vi "SpectralCurrent.vi"() -> ()   [LabVIEW 2009]
uses:
  <vilib>/Utility/file.llb/Write To Spreadsheet File (DBL).vi
  <vilib>/DAQmx/configure/timing.llb/DAQmx Timing (Sample Clock).vi
  <vilib>/DAQmx/create/channels.llb/DAQmx Create Channel (AI-Voltage-Basic).vi
  <vilib>/Utility/file.llb/Read From Spreadsheet File (DBL).vi
  <vilib>/DAQmx/read.llb/DAQmx Read (Analog 1D DBL 1Chan NSamp).vi
  <vilib>/Analysis/NI_AALBase.lvlib
panel:
  in  "Open Power Normalization Values Path":path
  in  "Normalize with file?":bool
  in  "Power Values Path":path
  out "Normalized Current":cluster{dbl[], dbl[]}(graph)
  in  "Save Current Path":path
  in  "Save Current?":bool
  out "Spectral Current":cluster{dbl[], dbl[]}(graph)
  in  "End Scan":bool
  out "Measuring Current":bool
  in  "Current":tag
  in  "Current Scan":bool
  in  "Exit":bool
  out "Scanning":bool
  in  "Scan Save Path":path
  in  "Save Power Scan?":bool
  out "Power Scan":cluster{dbl[], dbl[]}(graph)
  in  "Abort\n Scan":bool
  in  "Wavelength\n   Step Size":dbl=1.0 min=0.1 max=100.0
  in  "Starting\nWavelength":dbl=400.0 min=400.0 max=2500.0
  in  "Ending\nWavelength":dbl=500.0 min=451.0 max=2501.0
  in  "Step Time (sec)":dbl=1.0 min=0.1 max=10.0 step=0.1
  in  "Measurement Save Path":path
  in  "Save Measurement?":bool
  out "Power Measurement":dbl[](graph)
  out "Readout value":dbl format="%^#_9e"
  out "Readout string":string
  in  "Timeout [ms]":i32=1000
  out "New":bool
  out "ZeroValue":dbl
  out "RANG_Val":dbl
  out "RANG_lbl":string
  out "Rng":string
  out "AUTO?":bool
  in  "AUTO":bool=TRUE
  in  "Range":i16=1 min=1 max=6 step=1
  out "PM Error log":string
  in  "Beam\nDiameter (mm)":dbl=4.0 min=1.0 max=9.0 step=0.5
  in  "BWIn":u16(ring) caption="Bandwidth" items=["HIGH", "LOW"]
  in  "Averaging Rate":i32=300 min=33 max=5000 step=1
  in  "Zero?":bool
  in  "Stop Measurement":bool
  out "IDN String":string
  out "Sensor SN":string
  out "Sensor Name":string
  out "Incrementing Down":bool
  out "Changing Wavelength":bool
  out "Incrementing Up":bool
  in  "Increment":dbl=10.0 min=0.1 max=50.0
  in  "Target\nWavelength":dbl=400.0 min=400.0 max=3000.0
  out "Wavelength (nm)":dbl
  out "Turning Turret":bool
  out "Current Blaze":string caption="Grating Blaze"
  out "Grating Density":dbl
  out "Grating Index":i32
  in  "Select Grating Blaze":string(combo)
  out "error out":errorcluster
  out "Status":string
  out "Emulating":bool
  out "Initialized":bool
  in  "Force\nInitialization":bool
  in  "Mono ID":string(combo)
  out "Current UniqueID":string
  in  "Measure Power":bool
  in  "Initialize":bool
  in  "Switch Turret":bool
  in  "Scan":bool
  in  "Increment Down":bool
  in  "Increment Up":bool
  in  "Change Wavelength":bool
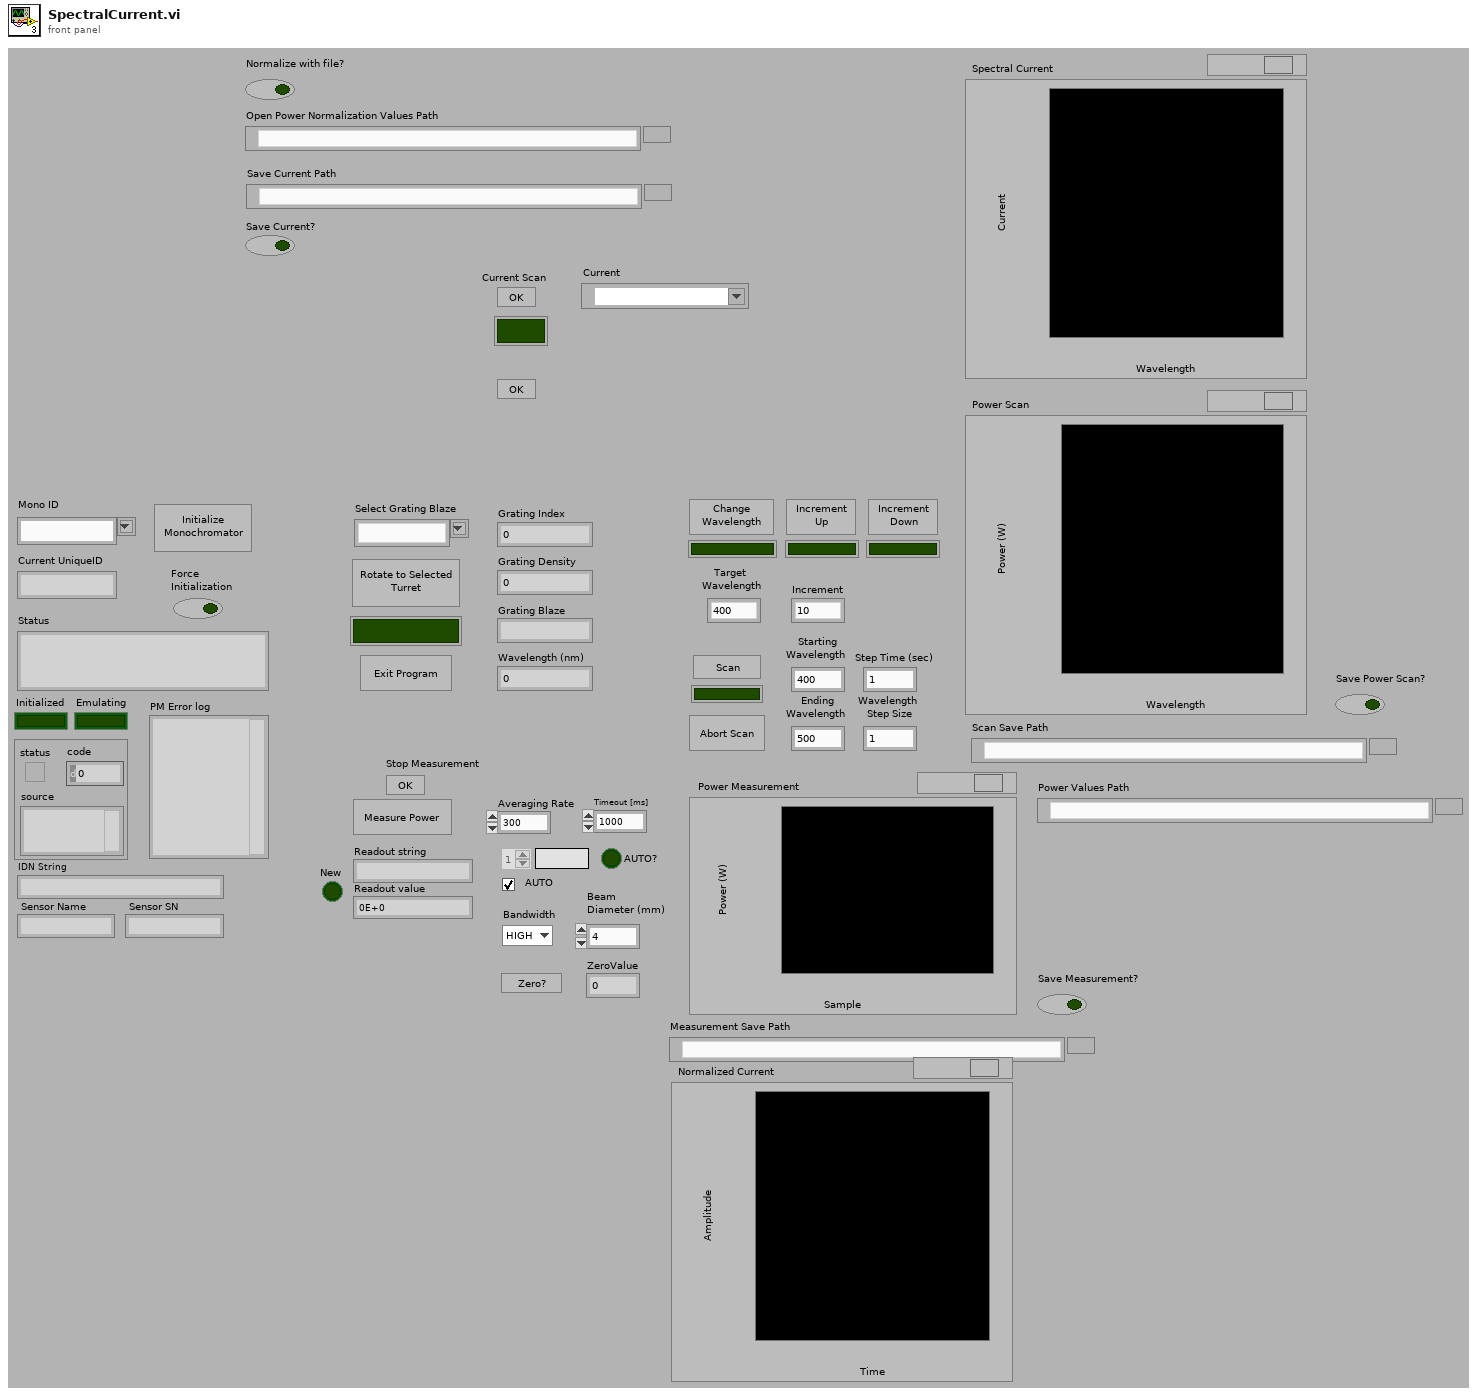
[diagram p1: front panel]
types:
  T1 = enum16{"0", "1", "2", "3", "4", "5", "6", "7", "8", "9"}
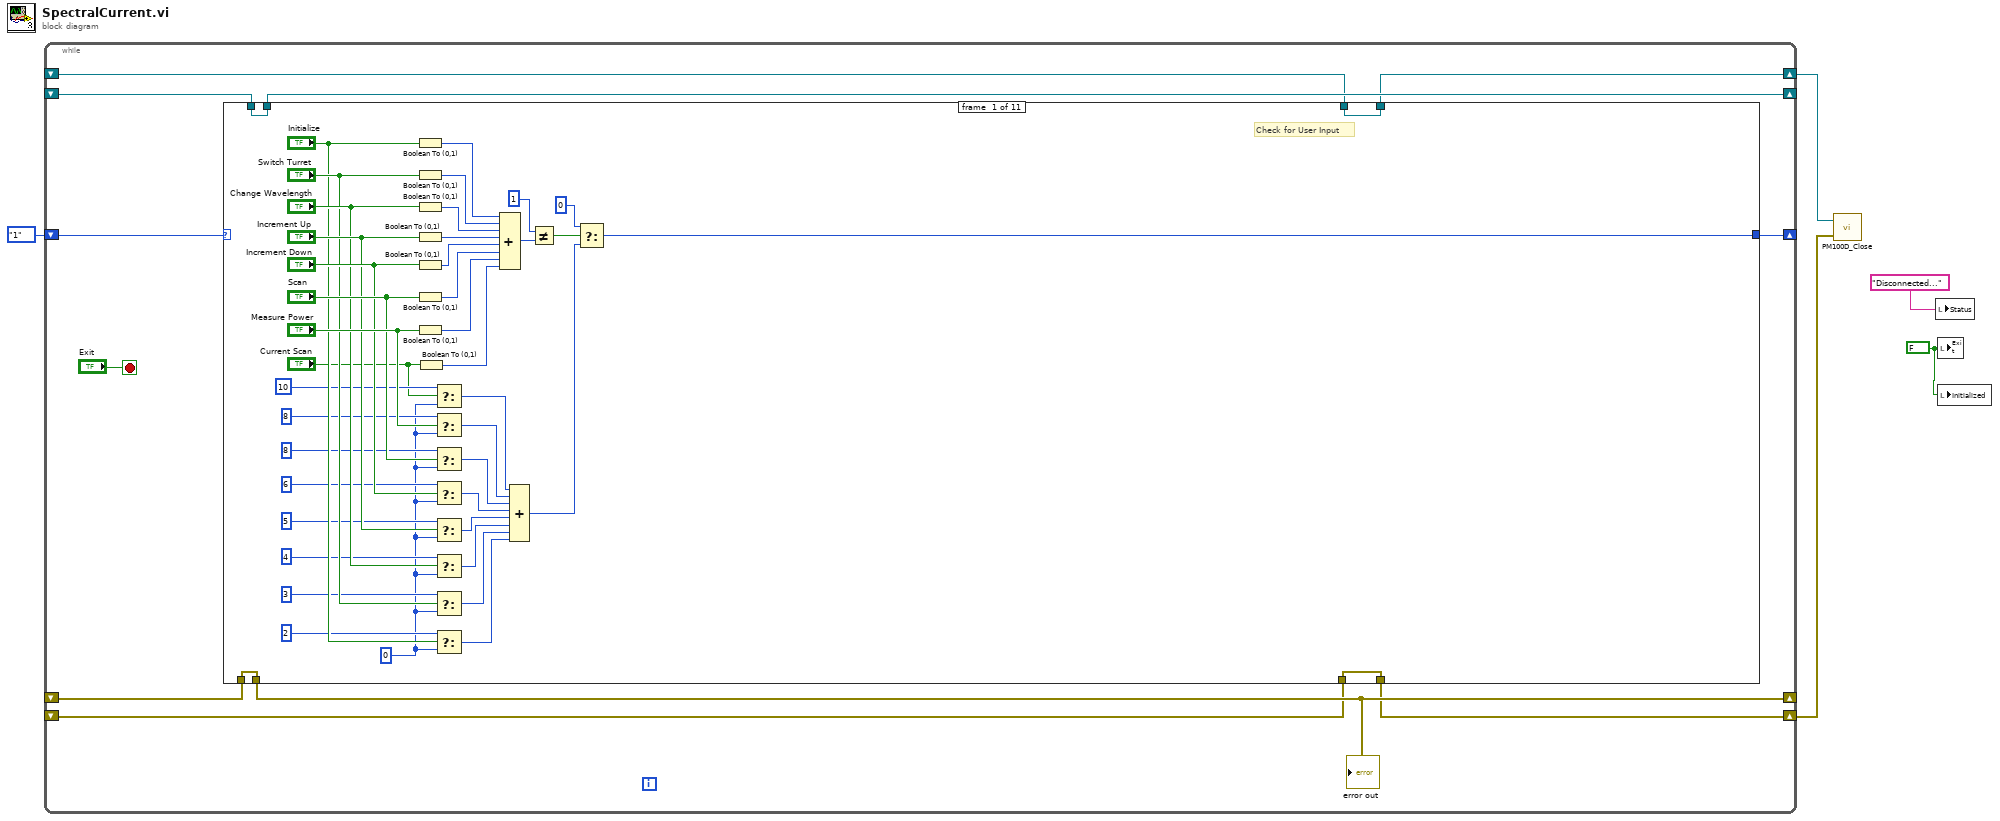
[diagram p0: block diagram]
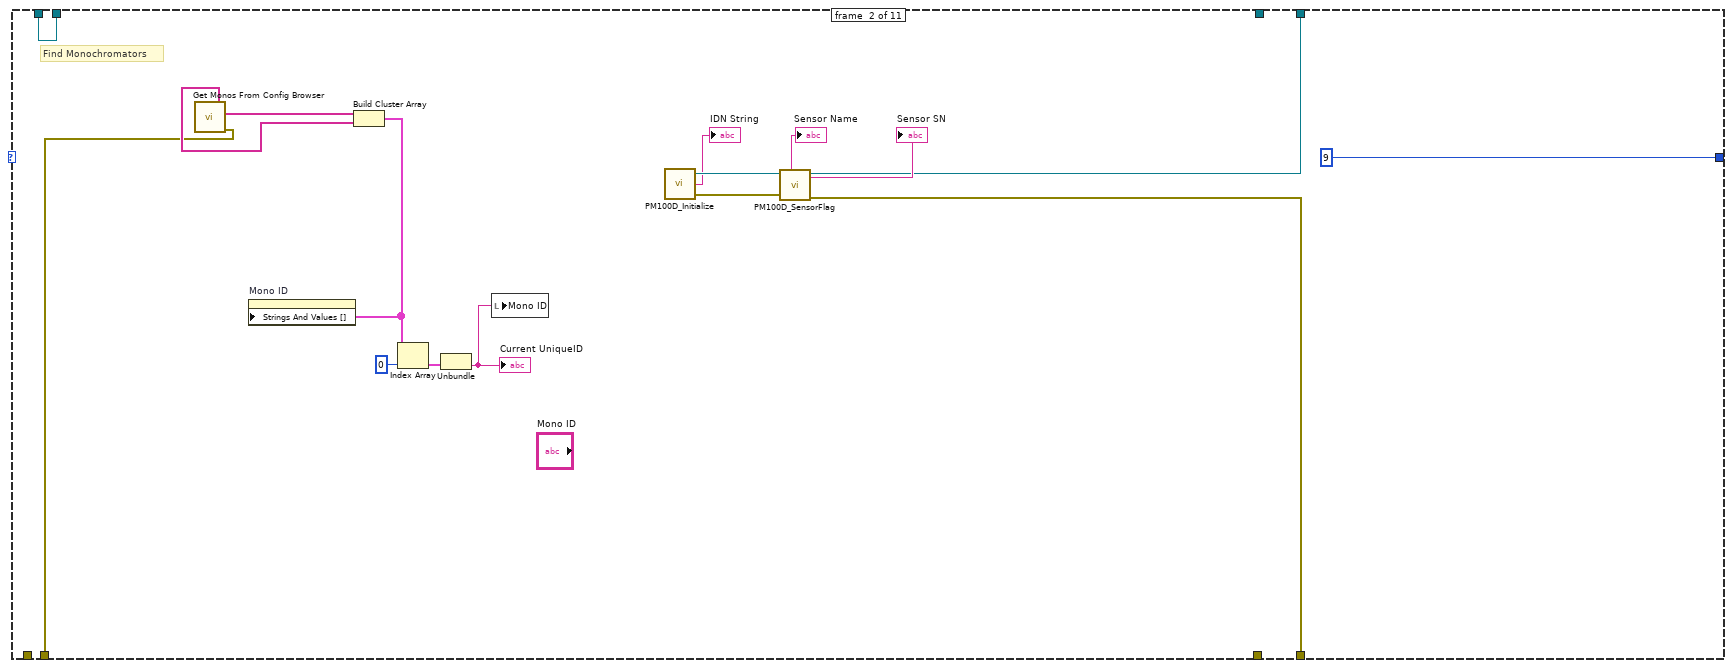
[diagram p2: hidden frame]
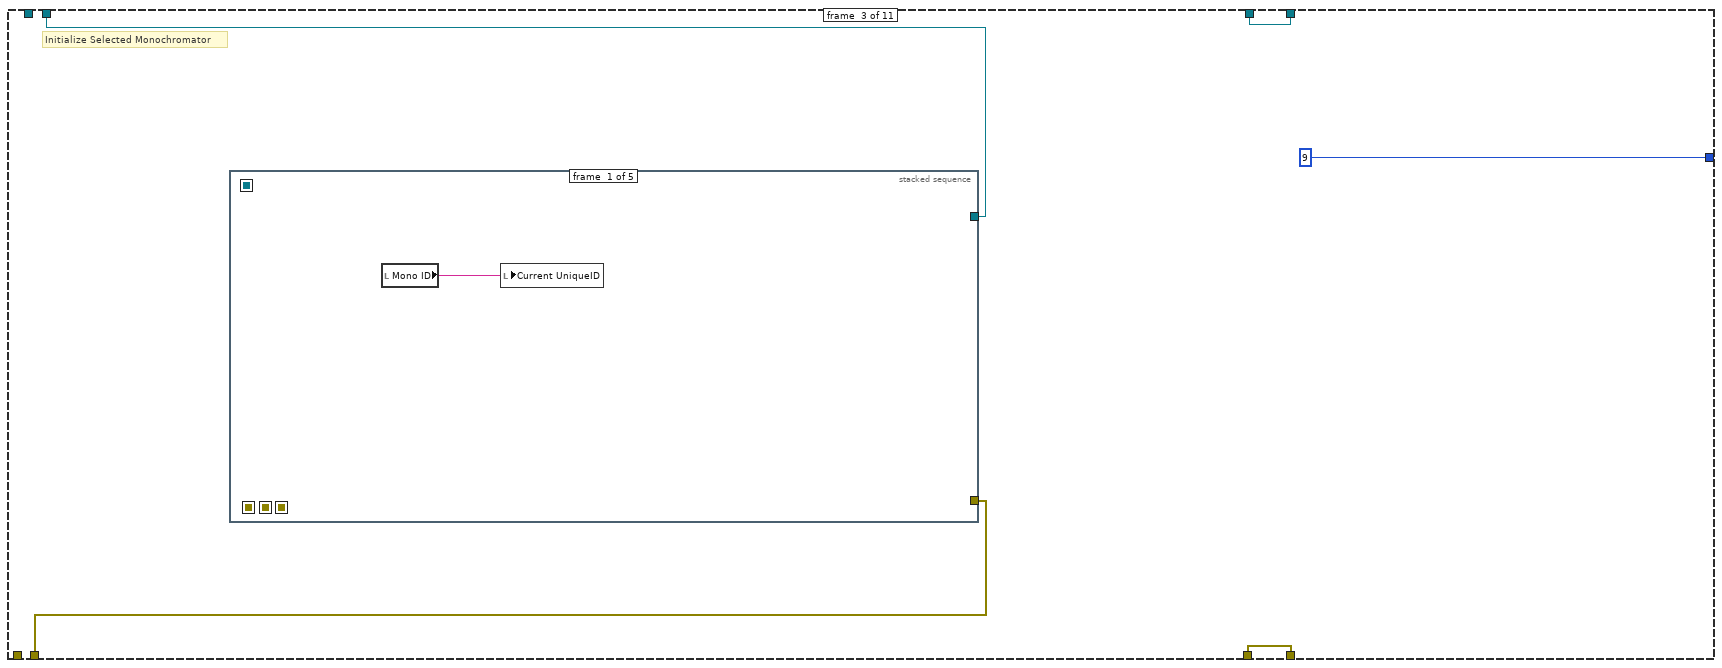
[diagram p3: hidden frame]
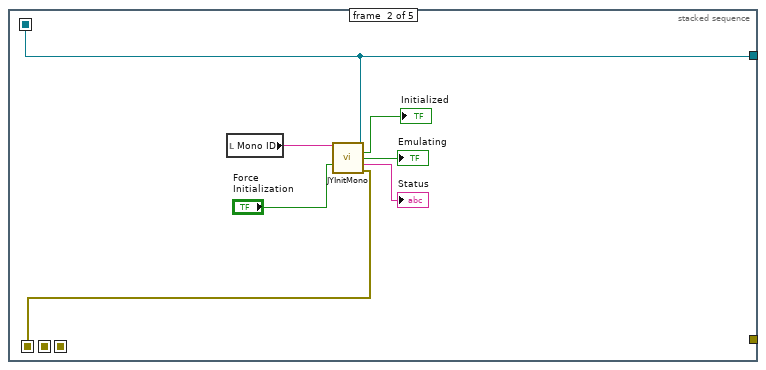
[diagram p4: hidden frame]
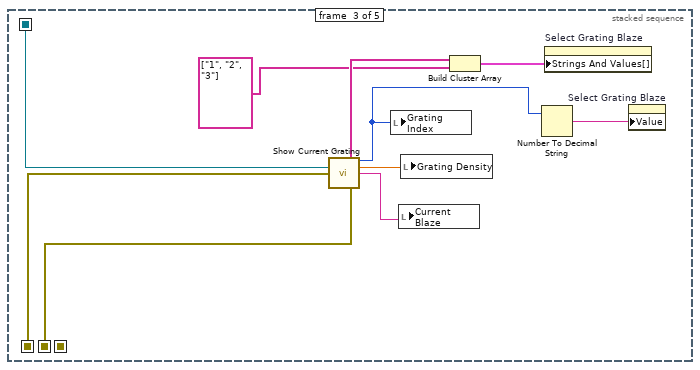
[diagram p5: hidden frame]
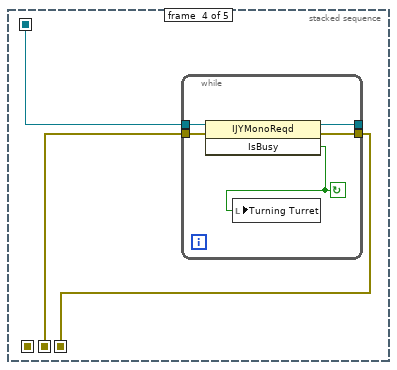
[diagram p6: hidden frame]
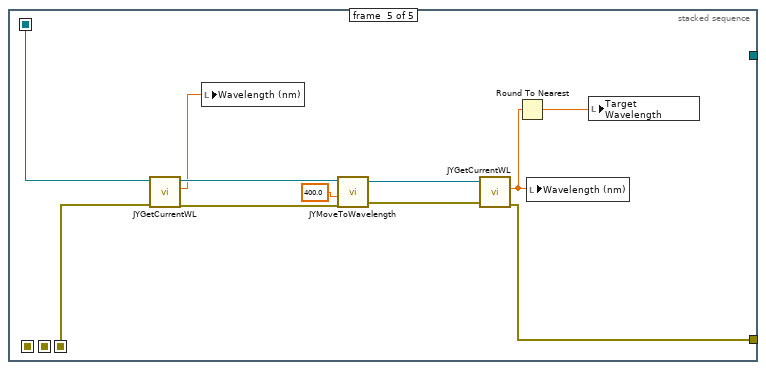
[diagram p7: hidden frame]
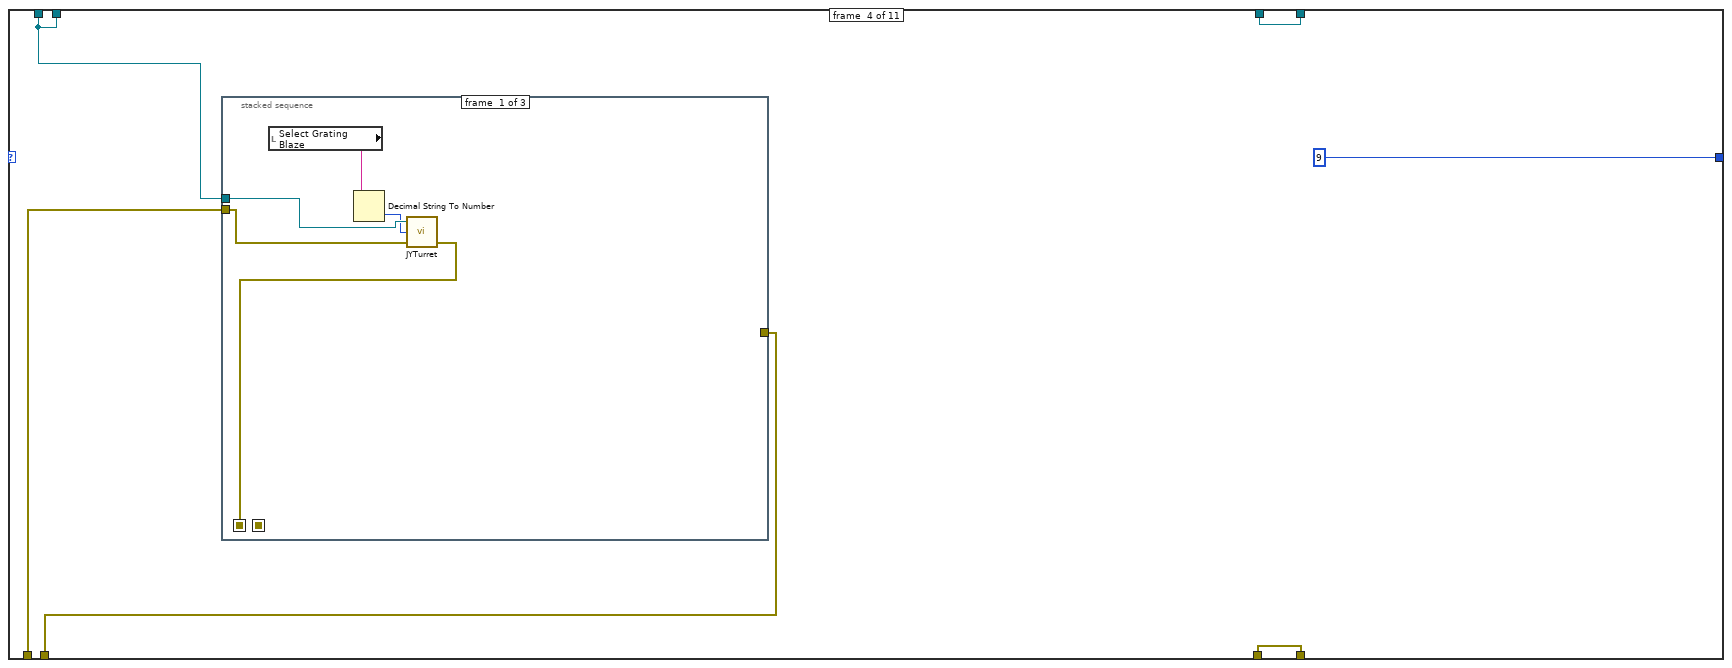
[diagram p8: hidden frame]
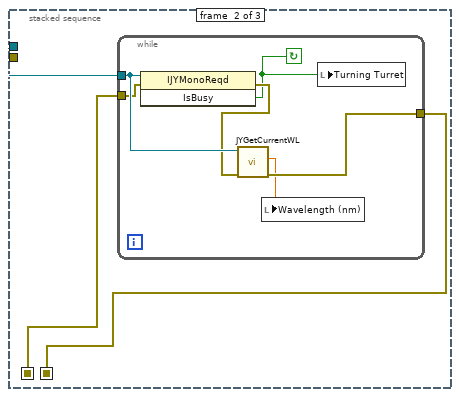
[diagram p9: hidden frame]
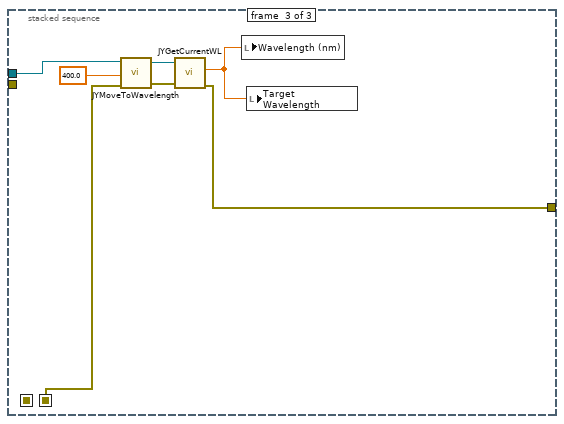
[diagram p10: hidden frame]
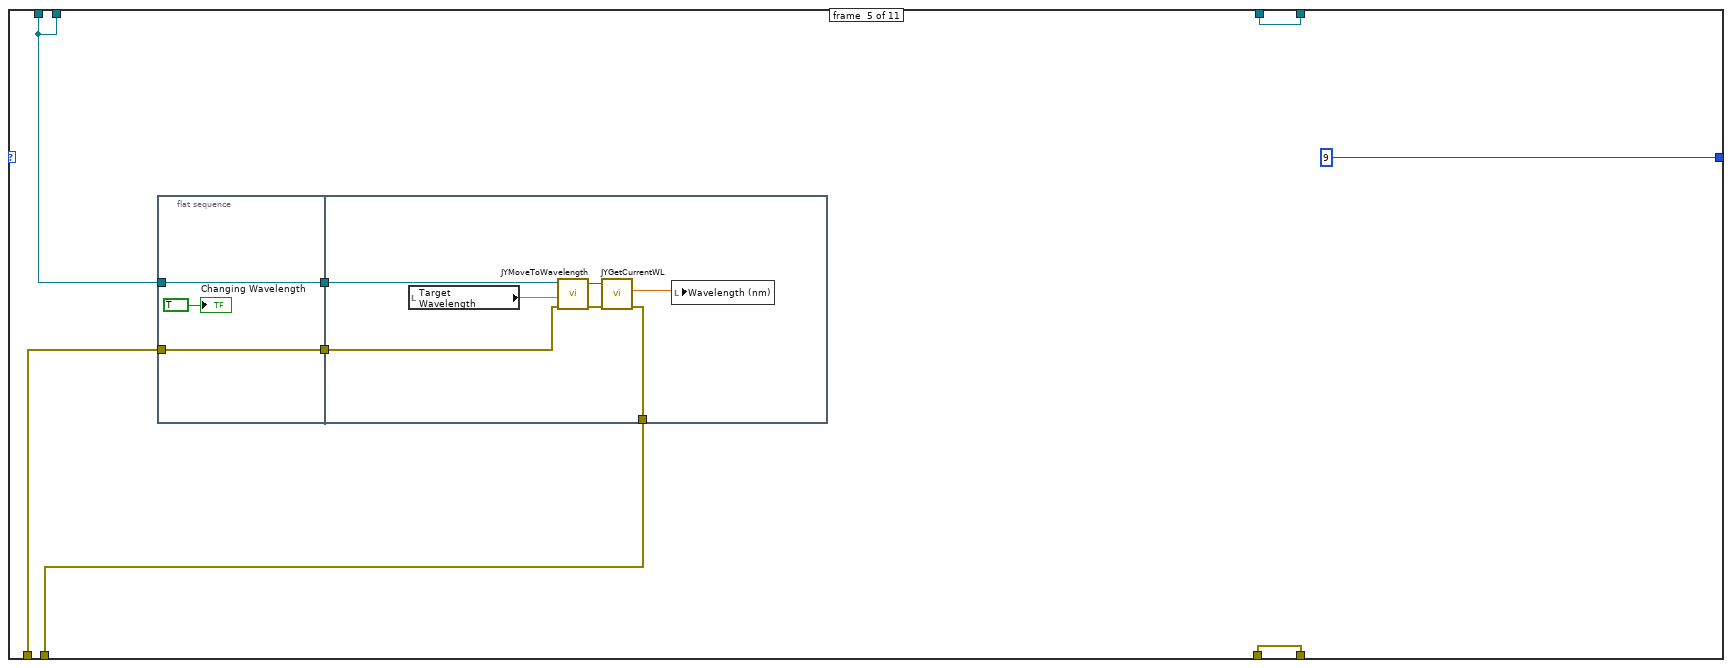
[diagram p11: hidden frame]
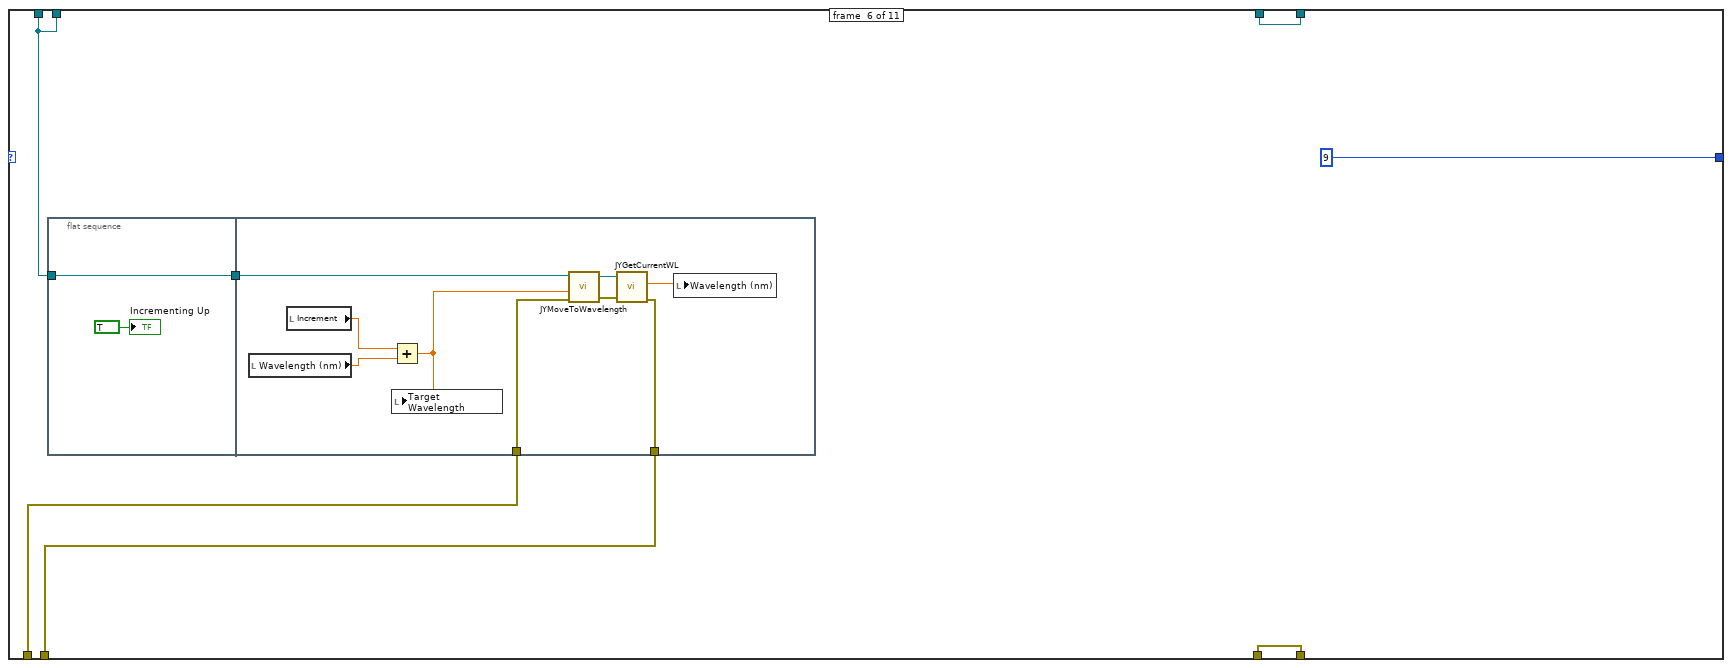
[diagram p12: hidden frame]
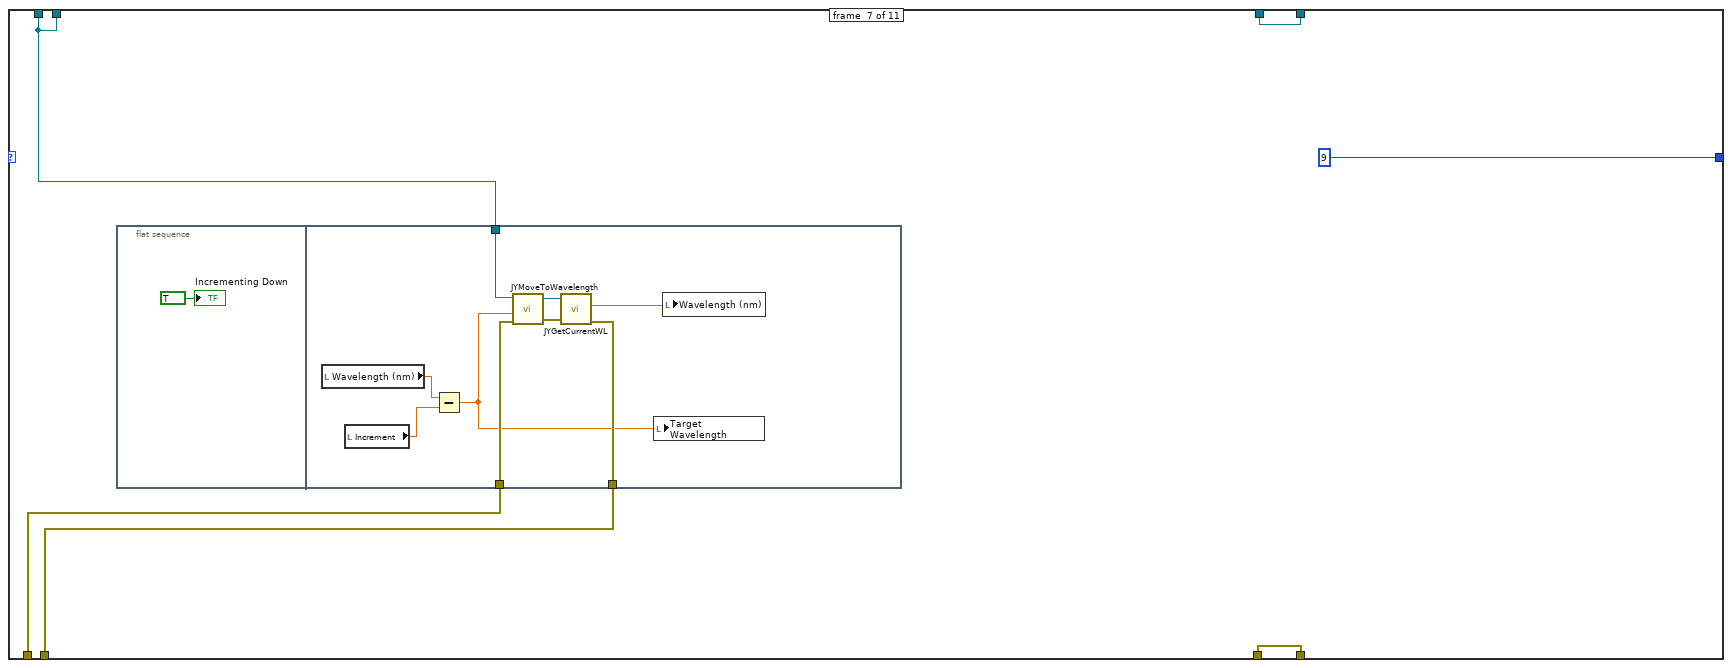
[diagram p13: hidden frame]
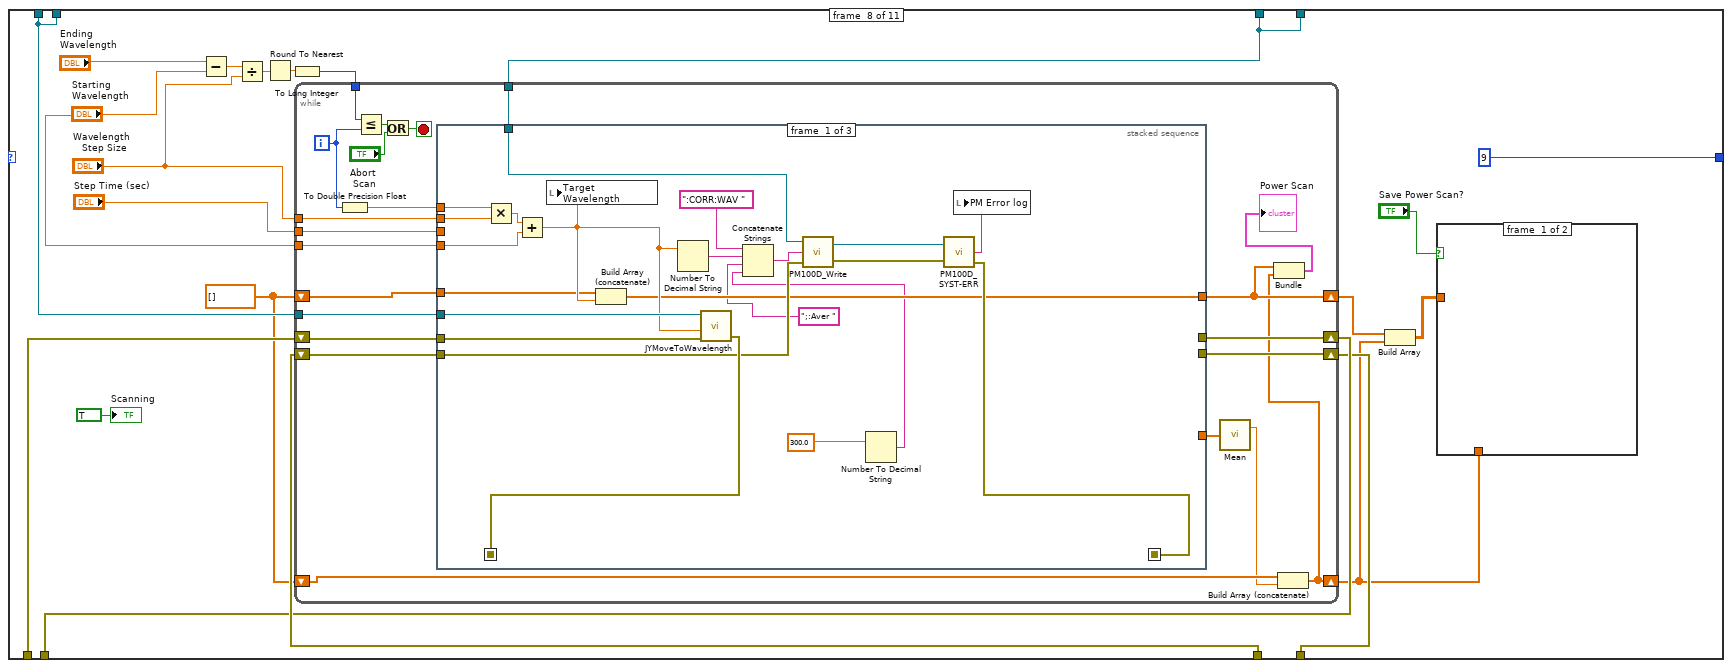
[diagram p14: hidden frame]
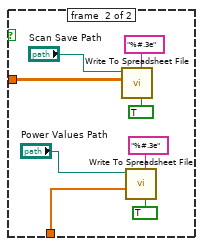
[diagram p15: hidden frame]
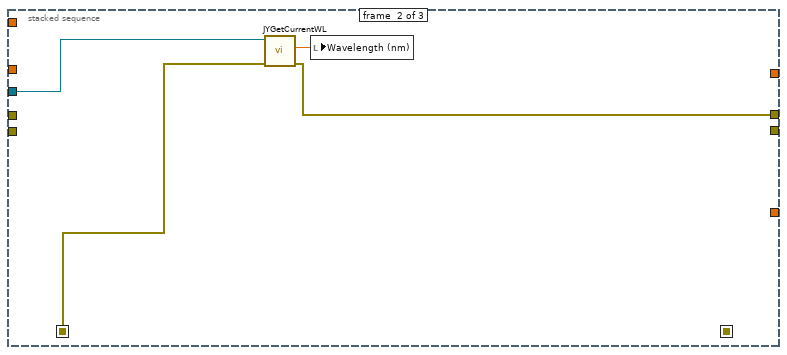
[diagram p16: hidden frame]
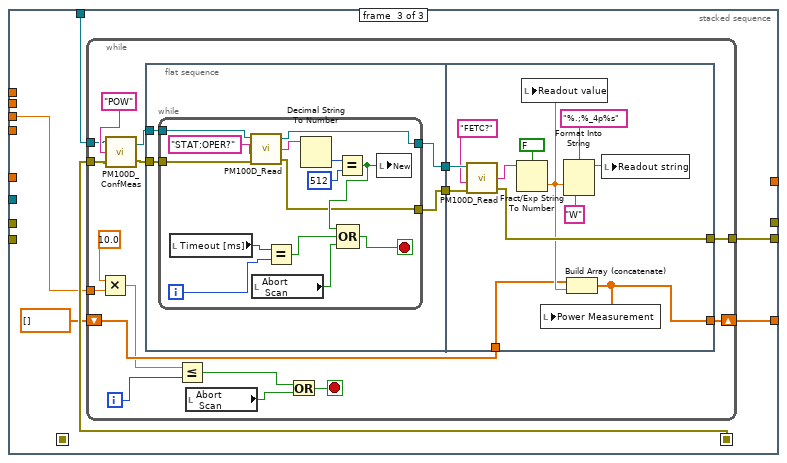
[diagram p17: hidden frame]
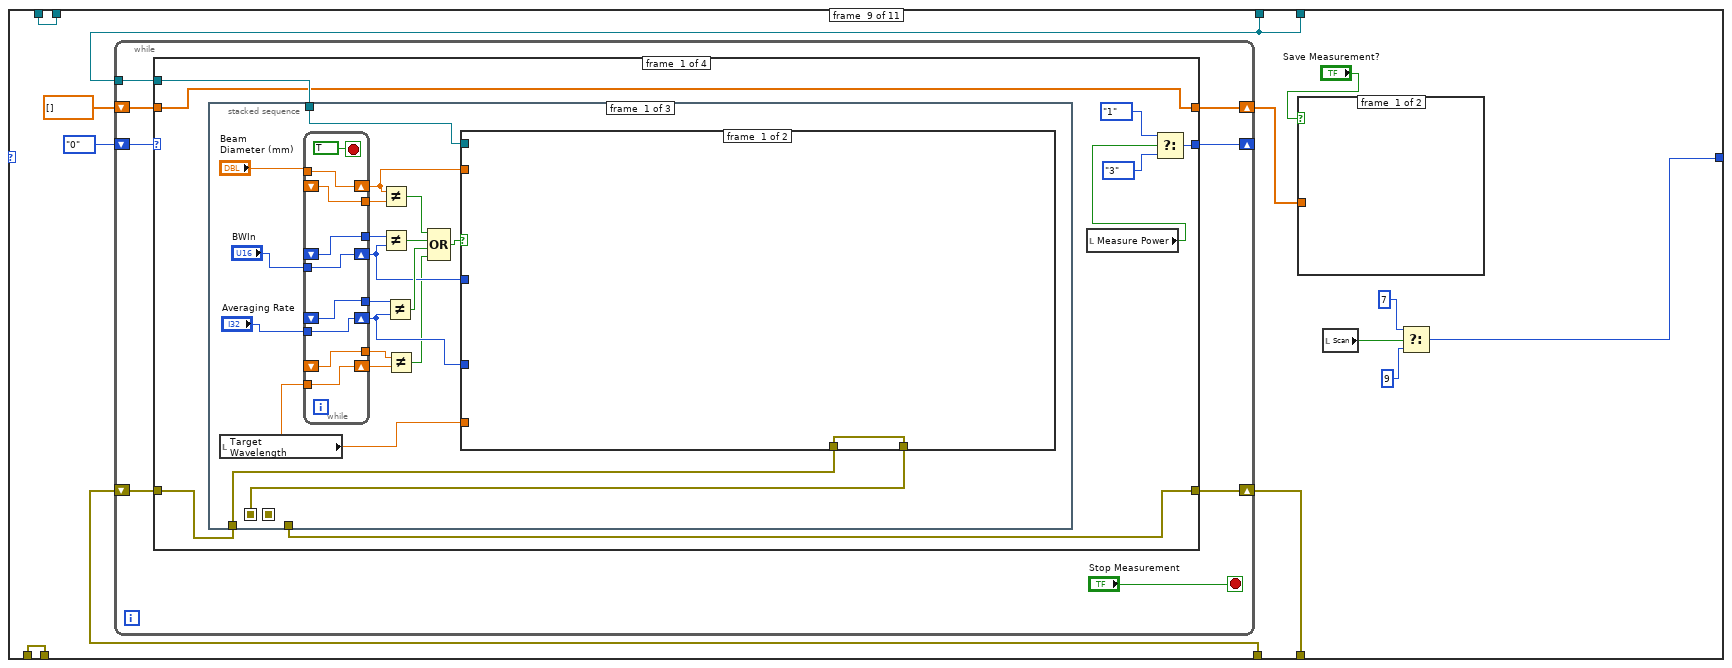
[diagram p18: hidden frame]
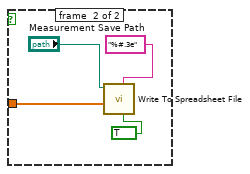
[diagram p19: hidden frame]
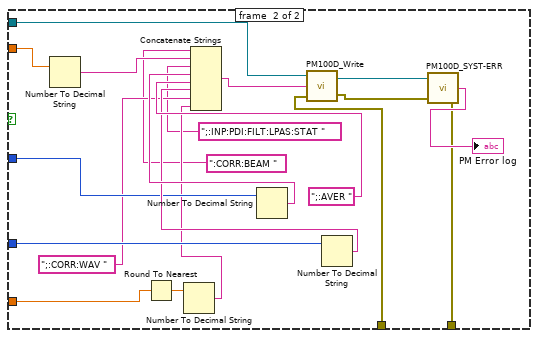
[diagram p20: hidden frame]
diagram:
  w1 = FALSE ("Exit")
  n1 = while {
    shift-right: [w16] -> _
    shift-left: T1."1" -> [w15]
    shift-right: [w14] -> _
    shift-left: _ -> [w13]
    shift-right: [w11] -> _
    shift-left: _ -> [w12]
    shift-right: [w10] -> w3
    shift-left: _ -> [w9]
    shift-right: [w8] -> w2
    shift-left: _ -> [w7]
    stop <- "Exit" stop-if-true
    n2 = case shown="10" w15 {
      tunnel: [w27 9 ("x") 9 ("x") 9 ("x") 9 ("x") 9 ("x") 9 ("x") 9 ("x") w327 0 ("x") 9 ("x")] -> w16
      tunnel: [w25 w68 w79 w121 w150 w167 w183 w210 w338 w509 w532] -> w14
      tunnel: [w24 w62 w78 w122 w149 w166 w185 w207 w339 w510 w528] -> w11
      tunnel: w13 -> [w25 w68 _ w121 w150 w167 w183 w210 w338 w509 w532]
      tunnel: w12 -> [w24 _ _ w120 w151 w168 w186 w209 w339 w510 w529]
      tunnel: [w23 w61 w77 w119 w146 w164 w182 w206 w334 w507 w523] -> w10
      tunnel: w9 -> [w23 _ w77 w119 w146 w164 w182 w208 w336 w507 w523]
      tunnel: [w22 w60 w76 w118 w145 w163 w181 w201 w335 w508 w522] -> w8
      tunnel: w7 -> [w22 _ w76 w118 w145 w163 w181 w201 w335 w508 w522]
      frame #0 {
        w19 = 0 ("x")
        # "Check for User Input"
        n3 = Boolean To (0,1)(Boolean="Initialize") -> (0, 1=w59:i16)
        n4 = Boolean To (0,1)(Boolean="Switch Turret") -> (0, 1=w58:i16)
        n5 = Boolean To (0,1)(Boolean="Change Wavelength") -> (0, 1=w57:i16)
        n6 = Boolean To (0,1)(Boolean="Increment Up") -> (0, 1=w56:i16)
        n7 = Boolean To (0,1)(Boolean="Increment Down") -> (0, 1=w55:i16)
        n8 = Boolean To (0,1)(Boolean="Scan") -> (0, 1=w54:i16)
        n9 = Boolean To (0,1)(Boolean="Measure Power") -> (0, 1=w53:i16)
        n10 = Boolean To (0,1)(Boolean="Current Scan") -> (0, 1=w21:i16)
        n11 = Select(t=10 ("x"), s="Current Scan", f=w19) -> (s? t:f=w20:i32)
        n12 = Select(t=8 ("x"), s="Measure Power", f=w19) -> (s? t:f=w43:i32)
        n13 = Select(t=8 ("x"), s="Scan", f=w19) -> (s? t:f=w42:i32)
        n14 = Select(t=6 ("x"), s="Increment Down", f=w19) -> (s? t:f=w41:i32)
        n15 = Select(t=5 ("x"), s="Increment Up", f=w19) -> (s? t:f=w40:i32)
        n16 = Select(t=4 ("x"), s="Change Wavelength", f=w19) -> (s? t:f=w39:i32)
        n17 = Select(t=3 ("x"), s="Switch Turret", f=w19) -> (s? t:f=w38:i32)
        n18 = Select(t=2 ("x"), s="Initialize", f=w19) -> (s? t:f=w37:i32)
        n19 = Compound Arithmetic op=ADD(w59, w58, w57, w56, w55, w54, w53, w21) -> (w52:i16)
        n20 = Compound Arithmetic op=ADD(w20, w43, w42, w41, w40, w39, w38, w37) -> (w28:i32)
        n21 = Not Equal?(x=i16 1, y=w52) -> (x != y?=w36:bool)
        n22 = Select(t=0 ("x"), s=w36, f=w28) -> (s? t:f=w27:i32)
      }
      frame #1 {
        # "Find Monochromators"
        n23 = call "Get Monos From Config Browser.vi"() -> ("UniqueIDs"=w72:string[], "Mono ID"=w71:string[], "error out"=w62:errorcluster)  [unwired: 3 in]
        n24 = Build Cluster Array(w71, w72) -> (w74:cluster{"String":string, "String":string}[])
        n25 = property on="Mono ID" class="CmbBox"("Strings And Values []"=w74) -> ()  [unwired: 2 in, 2 out]
        n26 = Index Array(array=w74, index=0) -> (element=w73:cluster{"String":string, "String":string})
        n27 = Unbundle(w73) -> ("String"=w69:string)  [unwired: 1 out]
        "Current UniqueID" <- w69
        n28 = local write "Mono ID"(w69) -> ()
        n29 = call "PM100D_Initialize.vi"() -> ("error out"=w66:errorcluster, "Instrument"=→"IDN String":string, "VISA out"=w67:refnum<visa-resource-name>)  [unwired: 2 in, 1 out]
        n30 = call "PM100D_SensorFlag.vi"("error in (no error)"=w66, "VISA in"=w67) -> ("error out"=w61:errorcluster, "VISA out"=w60:refnum<visa-resource-name>, "sn"=→"Sensor SN":string, "name"=→"Sensor Name":string)  [unwired: 2 in, 4 out]
      }
      frame #2 {
        # "Initialize Selected Monochromator"
        n31 = stacked-sequence {
          seq-local: [_ w83 _ _ _] -> [_ _ w98 _ _]
          seq-local: [_ w82 _ _ _] -> [_ _ w97 w100 w115]
          seq-local: [_ _ w93 _ _] -> [_ _ _ w101 _]
          seq-local: [_ _ _ w99 _] -> [_ _ _ _ w116]
          tunnel: [_ _ _ _ w107] -> w78
          tunnel: [_ w82 _ _ _] -> w79
          frame #0 {
            n32 = local read "Mono ID"() -> (w81:string)
            n33 = local write "Current UniqueID"(w81) -> ()
          }
          frame #1 {
            n34 = local read "Mono ID"() -> (w84:string)
            n35 = call "JYInitMono.vi"("Unique ID"=w84, "Force Init"="Force\nInitialization") -> ("Mono RefNum out"=w82:refnum<k7>, "Initialized"=→"Initialized":bool, "Emulating"=→"Emulating":bool, "Status"=→"Status":string, "error out"=w83:errorcluster)  [unwired: 9 in]
          }
          frame #2 {
            n36 = call "Show Current Grating.vi"("Refnum in"=w97, "error in (no error)"=w98) -> ("Blazes"=w96:string[], "Grating Index"=w91:i32, "Current Grating"=w89:dbl, "Current Blaze"=w90:string, "error out"=w93:errorcluster)  [unwired: 5 in, 4 out]
            n37 = local write "Grating Index"(w91) -> ()
            n38 = local write "Current Blaze"(w90) -> ()
            n39 = local write "Grating Density"(w89) -> ()
            n40 = Build Cluster Array(w96, string[] ["1", "2", "3"]) -> (w94:cluster{"String":string, string}[])
            n41 = Number To Decimal String(number=w91) -> (decimal integer string=w92:string)  [unwired: 1 in]
            n42 = property on="Select Grating Blaze" class="CmbBox"("Strings And Values[]"=w94) -> ()  [unwired: 2 in, 2 out]
            n43 = property on="Select Grating Blaze" class="CmbBox"("Value"=w92) -> ()  [unwired: 2 in, 2 out]
          }
          frame #3 {
            n44 = while {
              tunnel: w100 -> [w106]
              tunnel: w101 -> [w105]
              tunnel: [w104] -> _
              tunnel: [w103] -> w99
              stop <- w102 continue-if-true
              n45 = invoke class="IJYMonoReqd" method="IsBusy"(reference=w106, error in=w105) -> (reference out=w104:refnum<k7>, error out=w103:errorcluster, "IsBusy"=w102:bool)  [unwired: 1 in]
              n46 = local write "Turning Turret"(w102) -> ()
            }
          }
          frame #4 {
            n47 = call "JYGetCurrentWL.vi"("error in (no error)"=w116, "JYMONOLib.IJYMonoReqd"=w115) -> ("error out"=w111:errorcluster, "Current WL"=w108:dbl, "Mono Refnum Out"=w114:refnum<k7>)  [unwired: 6 in, 1 out]
            n48 = local write "Wavelength (nm)"(w108) -> ()
            n49 = call "JYMoveToWavelength.vi"("error in (no error)"=w111, "Target WL"=400.0, "RefNum In"=w114) -> ("error out"=w110:errorcluster, "Refnum Out"=w113:refnum<k7>)  [unwired: 1 in, 1 out]
            n50 = call "JYGetCurrentWL.vi"("error in (no error)"=w110, "JYMONOLib.IJYMonoReqd"=w113) -> ("error out"=w107:errorcluster, "Current WL"=w109:dbl)  [unwired: 6 in, 2 out]
            n51 = Round To Nearest(number=w109) -> (nearest integer value=w112:dbl)
            n52 = local write "Wavelength (nm)"(w109) -> ()
            n53 = local write "Target\nWavelength"(w112) -> ()
          }
        }
      }
      frame #3 {
        n54 = stacked-sequence {
          seq-local: [w126 _ _] -> [_ w130 _]
          seq-local: [_ w129 _] -> [_ _ w139]
          tunnel: w120 -> [w128 _ _]
          tunnel: w121 -> [w127 w131 w143]
          tunnel: [_ _ w138] -> w122
          frame #0 {
            n55 = local read "Select Grating Blaze"() -> (w124:string)
            n56 = Decimal String To Number(string=w124) -> (number=w125:i32)  [unwired: 2 in, 1 out]
            n57 = call "JYTurret.vi"("error in (no error)"=w128, "Grating Index"=w125, "RefNum In"=w127) -> ("error out"=w126:errorcluster)  [unwired: 2 out]
          }
          frame #1 {
            n58 = while {
              tunnel: w131 -> [w137]
              tunnel: w130 -> [w136]
              tunnel: [w134] -> w129
              stop <- w133 continue-if-true
              n59 = invoke class="IJYMonoReqd" method="IsBusy"(reference=w137, error in=w136) -> (error out=w135:errorcluster, "IsBusy"=w133:bool)  [unwired: 1 in, 1 out]
              n60 = call "JYGetCurrentWL.vi"("error in (no error)"=w135, "JYMONOLib.IJYMonoReqd"=w137) -> ("error out"=w134:errorcluster, "Current WL"=w132:dbl)  [unwired: 6 in, 2 out]
              n61 = local write "Wavelength (nm)"(w132) -> ()
              n62 = local write "Turning Turret"(w133) -> ()
            }
          }
          frame #2 {
            n63 = call "JYMoveToWavelength.vi"("error in (no error)"=w139, "Target WL"=400.0, "RefNum In"=w143) -> ("error out"=w141:errorcluster, "Refnum Out"=w142:refnum<k7>)  [unwired: 1 in, 1 out]
            n64 = call "JYGetCurrentWL.vi"("error in (no error)"=w141, "JYMONOLib.IJYMonoReqd"=w142) -> ("error out"=w138:errorcluster, "Current WL"=w140:dbl)  [unwired: 6 in, 2 out]
            n65 = local write "Wavelength (nm)"(w140) -> ()
            n66 = local write "Target\nWavelength"(w140) -> ()
          }
        }
      }
      frame #4 {
        n67 = flat-sequence {
          tunnel: w150 -> [w154]
          tunnel: w151 -> [w155]
          tunnel: [w155] -> w148
          tunnel: [w154] -> w147
          tunnel: [w156] -> w149
          tunnel: w148 -> [w159]
          tunnel: w147 -> [w158]
          frame #0 {
            "Changing Wavelength" <- TRUE
          }
          frame #1 {
            n68 = local read "Target\nWavelength"() -> (w162:dbl)
            n69 = call "JYMoveToWavelength.vi"("error in (no error)"=w159, "Target WL"=w162, "RefNum In"=w158) -> ("error out"=w161:errorcluster, "Refnum Out"=w160:refnum<k7>)  [unwired: 1 in, 1 out]
            n70 = call "JYGetCurrentWL.vi"("error in (no error)"=w161, "JYMONOLib.IJYMonoReqd"=w160) -> ("error out"=w156:errorcluster, "Current WL"=w157:dbl)  [unwired: 6 in, 2 out]
            n71 = local write "Wavelength (nm)"(w157) -> ()
          }
        }
      }
      frame #5 {
        n72 = flat-sequence {
          tunnel: w167 -> [w171]
          tunnel: [w171] -> w165
          tunnel: w168 -> [w178]
          tunnel: [w174] -> w166
          tunnel: w165 -> [w175]
          frame #0 {
            "Incrementing Up" <- TRUE
          }
          frame #1 {
            n73 = local read "Wavelength (nm)"() -> (w179:dbl)
            n74 = local read "Increment"() -> (w180:dbl)
            n75 = Add(x=w180, y=w179) -> (x+y=w173:dbl)
            n76 = local write "Target\nWavelength"(w173) -> ()
            n77 = call "JYMoveToWavelength.vi"("error in (no error)"=w178, "Target WL"=w173, "RefNum In"=w175) -> ("error out"=w177:errorcluster, "Refnum Out"=w176:refnum<k7>)  [unwired: 1 in, 1 out]
            n78 = call "JYGetCurrentWL.vi"("error in (no error)"=w177, "JYMONOLib.IJYMonoReqd"=w176) -> ("error out"=w174:errorcluster, "Current WL"=w172:dbl)  [unwired: 6 in, 2 out]
            n79 = local write "Wavelength (nm)"(w172) -> ()
          }
        }
      }
      frame #6 {
        n80 = flat-sequence {
          tunnel: w186 -> [w192]
          tunnel: w183 -> [w191]
          tunnel: [w190] -> w185
          frame #0 {
            "Incrementing Down" <- TRUE
          }
          frame #1 {
            n81 = local read "Wavelength (nm)"() -> (w194:dbl)
            n82 = local read "Increment"() -> (w193:dbl)
            n83 = Subtract(x=w194, y=w193) -> (x-y=w189:dbl)
            n84 = call "JYMoveToWavelength.vi"("error in (no error)"=w192, "Target WL"=w189, "RefNum In"=w191) -> ("error out"=w196:errorcluster, "Refnum Out"=w195:refnum<k7>)  [unwired: 1 in, 1 out]
            n85 = call "JYGetCurrentWL.vi"("error in (no error)"=w196, "JYMONOLib.IJYMonoReqd"=w195) -> ("error out"=w190:errorcluster, "Current WL"=w188:dbl)  [unwired: 6 in, 2 out]
            n86 = local write "Target\nWavelength"(w189) -> ()
            n87 = local write "Wavelength (nm)"(w188) -> ()
          }
        }
      }
      frame #7 {
        w205 = dbl[] []
        n88 = Subtract(x="Ending\nWavelength", y="Starting\nWavelength") -> (x-y=w215:dbl)
        n89 = Divide(x=w215, y="Wavelength\n   Step Size") -> (x/y=w199:dbl)
        n90 = Round To Nearest(number=w199) -> (nearest integer value=w198:dbl)
        n91 = To Long Integer(number=w198) -> (32bit integer=w214:i32)
        n92 = while {
          tunnel: w214 -> [w247]
          tunnel: "Wavelength\n   Step Size" -> [w243]
          tunnel: "Step Time (sec)" -> [w242]
          tunnel: "Starting\nWavelength" -> [w241]
          tunnel: w210 -> [w238]
          shift-right: [w228] -> w204
          shift-left: w205 -> [w235]
          shift-right: [w234] -> w207
          shift-left: w209 -> [w237]
          tunnel: w201 -> [w233]
          shift-right: [w232] -> w206
          shift-left: w208 -> [w236]
          shift-right: [w227] -> w197
          shift-left: w205 -> [w230]
          i -> [w240]
          stop <- w245 stop-if-true
          n93 = To Double Precision Float(number=w240) -> (double precision float=w239:dbl)
          n94 = Less Or Equal?(x=w247, y=w240) -> (x <= y?=w246:bool)
          n95 = Or(x=w246, y="Abort\n Scan") -> (x .or. y?=w245:bool)
          n96 = stacked-sequence {
            seq-local: [w259 _ _] -> [_ w272 _]
            seq-local: [w257 _ _] -> [_ _ w279]
            tunnel: w243 -> [w265 _ _]
            tunnel: w242 -> [_ _ w275]
            tunnel: w241 -> [w262 _ _]
            tunnel: w239 -> [w264 _ _]
            tunnel: w238 -> [w261 w273 _]
            tunnel: w237 -> [w260 _ _]
            tunnel: w236 -> [w258 _ _]
            tunnel: w235 -> [w255 _ _]
            tunnel: [w254 _ _] -> w228
            tunnel: [_ w271 _] -> w234
            tunnel: w233 -> [w249 _ w278]
            tunnel: [_ _ w277] -> w232
            tunnel: [_ _ w274] -> w231
            frame #0 {
              n97 = Multiply(x=w264, y=w265) -> (x*y=w263:dbl)
              n98 = Add(x=w263, y=w262) -> (x+y=w256:dbl)
              n99 = local write "Target\nWavelength"(w256) -> ()
              n100 = Build Array (concatenate)(w255, w256) -> (w254:dbl[])
              n101 = Number To Decimal String(number=w256) -> (decimal integer string=w268:string)  [unwired: 1 in]
              n102 = call "JYMoveToWavelength.vi"("error in (no error)"=w260, "Target WL"=w256, "RefNum In"=w261) -> ("error out"=w259:errorcluster)  [unwired: 1 in, 2 out]
              n103 = Number To Decimal String(number=300.0 ("y")) -> (decimal integer string=w251:string)  [unwired: 1 in]
              n104 = Concatenate Strings(":CORR:WAV " ("string"), w268, ";:Aver " ("string"), w251) -> (w269:string)
              n105 = call "PM100D_Write.vi"("error in (no error)"=w258, "Command"=w269, "VISA in"=w249) -> ("error out"=w252:errorcluster, "VISA out"=w253:refnum<visa-resource-name>)
              n106 = call "PM100D_SYST-ERR.vi"("error out 2"=w252, "VISA In"=w253) -> ("error out"=w257:errorcluster, "Error"=w266:string)  [unwired: 1 in, 1 out]
              n107 = local write "PM Error log"(w266) -> ()
            }
            frame #1 {
              n108 = call "JYGetCurrentWL.vi"("error in (no error)"=w272, "JYMONOLib.IJYMonoReqd"=w273) -> ("error out"=w271:errorcluster, "Current WL"=w270:dbl)  [unwired: 6 in, 2 out]
              n109 = local write "Wavelength (nm)"(w270) -> ()
            }
            frame #2 {
              n110 = while {
                tunnel: w279 -> [w296]
                tunnel: w278 -> [w293]
                tunnel: [w289] -> w277
                shift-right: [w287] -> w274
                shift-left: dbl[] [] -> [w288]
                tunnel: w275 -> [w282]
                i -> [w283]
                stop <- w286 stop-if-true
                n111 = Multiply(x=10.0 ("y"), y=w282) -> (x*y=w280:dbl)
                n112 = call "PM100D_ConfMeas.vi"("error in"=w296, "Conf:"="POW" ("Command"), "VISA In"=w293) -> ("error out"=w295:errorcluster, "dup VISA session"=w292:refnum<visa-resource-name>)
                n113 = flat-sequence {
                  tunnel: w295 -> [w300]
                  tunnel: w292 -> [w299]
                  tunnel: [w298] -> w291
                  tunnel: [w297] -> w290
                  tunnel: w291 -> [w323]
                  tunnel: w290 -> [w322]
                  tunnel: [w318] -> w289
                  tunnel: w288 -> [w316]
                  tunnel: [w315] -> w287
                  frame #0 {
                    n114 = while {
                      tunnel: w300 -> [w304]
                      tunnel: [w303] -> w297
                      tunnel: w299 -> [w302]
                      tunnel: [w301] -> w298
                      i -> [w312]
                      stop <- w314 stop-if-true
                      n115 = local read "Timeout [ms]"() -> (w311:i32)
                      n116 = call "PM100D_Read.vi"("error in (no error)"=w304, "Command"="STAT:OPER?", "VISA in"=w302) -> ("error out"=w303:errorcluster, "ReadValue"=w306:string, "VISA out"=w301:refnum<visa-resource-name>)  [unwired: 1 in]
                      n117 = local read "Abort\n Scan"() -> (w313:bool)
                      n118 = Equal?(x=w311, y=w312) -> (x = y?=w310:bool)
                      n119 = Decimal String To Number(string=w306) -> (number=w309:i32)  [unwired: 2 in, 1 out]
                      n120 = Equal?(x=w309, y=512) -> (x = y?=w307:bool)
                      n121 = Compound Arithmetic op=OR(w307, w310, w313) -> (w314:bool)
                      n122 = local write "New"(w307) -> ()
                    }
                  }
                  frame #1 {
                    n123 = call "PM100D_Read.vi"("error in (no error)"=w322, "Command"="FETC?", "VISA in"=w323) -> ("error out"=w318:errorcluster, "ReadValue"=w320:string)  [unwired: 1 in, 1 out]
                    n124 = Fract/Exp String To Number(use system decimal point (T)=FALSE, string=w320) -> (number=w317:dbl)  [unwired: 2 in, 1 out]
                    n125 = local write "Readout value"(w317) -> ()
                    n126 = Format Into String(format string="%.;%_4p%s", w317, "W") -> (resulting string=w319:string)  [unwired: 2 in, 1 out]
                    n127 = Build Array (concatenate)(w316, w317) -> (w315:dbl[])
                    n128 = local write "Power Measurement"(w315) -> ()
                    n129 = local write "Readout string"(w319) -> ()
                  }
                }
                n130 = Less Or Equal?(x=w280, y=w283) -> (x <= y?=w285:bool)
                n131 = local read "Abort\n Scan"() -> (w284:bool)
                n132 = Or(x=w285, y=w284) -> (x .or. y?=w286:bool)
              }
            }
          }
          n133 = call <vilib>:"Mean.vi"("X"=w231) -> ("mean"=w229:dbl)  [unwired: 1 out]
          n134 = Build Array (concatenate)(w230, w229) -> (w227:dbl[])
          n135 = Bundle(w228, w227) -> (→"Power Scan":cluster{dbl[], dbl[]})  [unwired: 1 in]
        }
        n136 = Build Array(w204, w197) -> (w203:dbl[][])
        n137 = case shown="True" "Save Power Scan?" {
          tunnel: w203 -> [_ w222]
          tunnel: w197 -> [_ w218]
          frame #0 {
          }
          frame #1 {
            n138 = call-poly <vilib>:"Write To Spreadsheet File.vi"("transpose? (no:F)"=TRUE, "format (%.3f)"="%#.3e", "2D data"=w222, "file path (dialog if empty)"="Scan Save Path") -> ()  [unwired: 4 in, 1 out]
            n139 = call-poly <vilib>:"Write To Spreadsheet File.vi"("transpose? (no:F)"=TRUE, "format (%.3f)"="%#.3e", "1D data"=w218, "file path (dialog if empty)"="Power Values Path") -> ()  [unwired: 4 in, 1 out]
          }
        }
        "Scanning" <- TRUE ("Scanning")
      }
      frame #8 {
        n140 = while {
          shift-right: [w350] -> _
          shift-left: enum16{"0", "1", "2", "3"}."0" -> [w351]
          shift-right: [w347] -> w334
          shift-left: w336 -> [w349]
          tunnel: w335 -> [w348]
          shift-right: [w345] -> w331
          shift-left: dbl[] [] -> [w346]
          stop <- "Stop Measurement" stop-if-true
          n141 = case shown="\"0\", Default" w351 {
            tunnel: [w355 w472 enum16{"0", "1", "2", "3"}."0" enum16{"0", "1", "2", "3"}."0"] -> w350
            tunnel: w349 -> [w359 w470 w494 w503]
            tunnel: w348 -> [w358 w469 w495 _]
            tunnel: [w357 w467 w493 w503] -> w347
            tunnel: w346 -> [w356 w466 w490 w504]
            tunnel: [w356 w466 w489 w504] -> w345
            frame #0 {
              n142 = stacked-sequence {
                seq-local: [w366 _ _] -> [_ w412 _]
                seq-local: [_ w410 _] -> [_ _ w454]
                tunnel: w359 -> [w367 _ _]
                tunnel: w358 -> [w365 w411 w452]
                tunnel: [_ _ w453] -> w357
                frame #0 {
                  n143 = local read "Target\nWavelength"() -> (w360:dbl)
                  n144 = while {
                    shift-right: [w408] -> w368
                    shift-left: _ -> [w407]
                    shift-right: [w404] -> w369
                    shift-left: _ -> [w403]
                    shift-right: [w406] -> w364
                    shift-left: _ -> [w405]
                    tunnel: "Beam\nDiameter (mm)" -> [w408]
                    tunnel: [w407] -> w379
                    tunnel: "Averaging Rate" -> [w406]
                    tunnel: [w405] -> w378
                    tunnel: "BWIn" -> [w404]
                    tunnel: [w403] -> w370
                    shift-right: [w402] -> w362
                    shift-left: _ -> [w401]
                    tunnel: w360 -> [w402]
                    tunnel: [w401] -> w363
                    stop <- TRUE stop-if-true
                  }
                  n145 = Not Equal?(x=w368, y=w379) -> (x != y?=w375:bool)
                  n146 = Not Equal?(x=w370, y=w369) -> (x != y?=w376:bool)
                  n147 = Not Equal?(x=w378, y=w364) -> (x != y?=w377:bool)
                  n148 = Not Equal?(x=w363, y=w362) -> (x != y?=w361:bool)
                  n149 = Compound Arithmetic op=OR(w375, w376, w377, w361) -> (w374:bool)
                  n150 = case shown="True" w374 {
                    tunnel: w364 -> [_ w392]
                    tunnel: w369 -> [_ w391]
                    tunnel: w368 -> [_ w390]
                    tunnel: w367 -> [w380 w389]
                    tunnel: [w380 w388] -> w366
                    tunnel: w365 -> [_ w387]
                    tunnel: w360 -> [_ w383]
                    frame #0 {
                    }
                    frame #1 {
                      n151 = Number To Decimal String(number=w390) -> (decimal integer string=w393:string)  [unwired: 1 in]
                      n152 = Round To Nearest(number=w383) -> (nearest integer value=w386:dbl)
                      n153 = Number To Decimal String(number=w386) -> (decimal integer string=w384:string)  [unwired: 1 in]
                      n154 = Number To Decimal String(number=w391) -> (decimal integer string=w397:string)  [unwired: 1 in]
                      n155 = Number To Decimal String(number=w392) -> (decimal integer string=w394:string)  [unwired: 1 in]
                      n156 = Concatenate Strings(":CORR:BEAM " ("string"), w393, ";:INP:PDI:FILT:LPAS:STAT ", w397, ";:AVER " ("string"), w394, ";:CORR:WAV " ("string"), w384) -> (w400:string)
                      n157 = call "PM100D_Write.vi"("error in (no error)"=w389, "Command"=w400, "VISA in"=w387) -> ("error out"=w398:errorcluster, "VISA out"=w399:refnum<visa-resource-name>)
                      n158 = call "PM100D_SYST-ERR.vi"("error out 2"=w398, "VISA In"=w399) -> ("error out"=w388:errorcluster, "Error"=→"PM Error log":string)  [unwired: 1 in, 1 out]
                    }
                  }
                }
                frame #1 {
                  n159 = while {
                    shift-right: [w449] -> w413
                    shift-left: _ -> [w448]
                    shift-right: [w451] -> w414
                    shift-left: _ -> [w450]
                    tunnel: "AUTO" -> [w451]
                    tunnel: [w450] -> w420
                    tunnel: "Range" -> [w449]
                    tunnel: [w448] -> w417
                    stop <- TRUE stop-if-true
                  }
                  n160 = Not Equal?(x=w414, y=w420) -> (x != y?=w419:bool)
                  n161 = Not Equal?(x=w413, y=w417) -> (x != y?=w416:bool)
                  n162 = Or(x=w419, y=w416) -> (x .or. y?=w415:bool)
                  n163 = case shown="False" w415 {
                    tunnel: w414 -> [_ w429]
                    tunnel: w413 -> [_ w428]
                    tunnel: w411 -> [_ w426]
                    tunnel: [w422 w424] -> w410
                    tunnel: w412 -> [w422 w423]
                    frame #0 {
                    }
                    frame #1 {
                      n164 = Decrement(x=w428) -> (x-1=w436:i16)
                      n165 = call "PM100D_Ranging.vi"("VISA in"=w426, "Index"=w436, "AUTO"=w429, "error in (no error)"=w423, "Unit"="POW") -> ("SensType"=w435:i32, "AUTO?"=→"AUTO?":bool, "RANG_Val"=→"RANG_Val":dbl, "RANG_lbl"=w444:string, "error out"=w424:errorcluster)  [unwired: 3 in, 3 out]
                      "RANG_lbl" <- w444
                      n166 = Equal?(x=w435, y=1) -> (x = y?=w440:bool)
                      n167 = Equal?(x=w435, y=3) -> (x = y?=w430:bool)
                      n168 = Select(t=2, s=w429, f=0) -> (s? t:f=w442:i32)
                      n169 = Select(t=6, s=w440, f=4) -> (s? t:f=w441:i32)
                      n170 = Concatenate Strings(w444, "W") -> (→"Rng":string)
                      n171 = Not(x=w430) -> (.not. x?=w431:bool)
                      n172 = property on="Range" class="DigNum (strict)"("Disabled"=w442, "Maximum"=w441) -> ()  [unwired: 2 in, 2 out]
                      n173 = property on="AUTO" class="Bool (strict)"("Visible"=w431) -> ()  [unwired: 2 in, 2 out]
                    }
                  }
                }
                frame #2 {
                  n174 = case shown="False" "Zero?" {
                    tunnel: w452 -> [_ w463]
                    tunnel: w454 -> [w456 w461]
                    tunnel: [w456 w460] -> w453
                    tunnel: w452 -> [_ w459]
                    frame #0 {
                    }
                    frame #1 {
                      n175 = call "PM100D_Zeroing.vi"("VISA In"=w463) -> ("ZeroValue"=→"ZeroValue":dbl)  [unwired: 4 in]
                      n176 = call "PM100D_SYST-ERR.vi"("error out 2"=w461, "VISA In"=w459) -> ("error out"=w460:errorcluster, "Error"=w458:string)  [unwired: 1 in, 1 out]
                      n177 = local write "PM Error log"(w458) -> ()
                      n178 = local write "Zero?"(FALSE ("Zero?")) -> ()
                    }
                  }
                }
              }
              n179 = local read "Measure Power"() -> (w354:bool)
              n180 = Select(t=enum16{"0", "1", "2", "3"}."1", s=w354, f=enum16{"0", "1", "2", "3"}."3") -> (s? t:f=w355:enum16{"0", "1", "2", "3"})
            }
            frame #1 {
              n181 = call "PM100D_ConfMeas.vi"("error in"=w470, "Conf:"="POW" ("Command"), "VISA In"=w469) -> ("error out"=w468:errorcluster)  [unwired: 1 out]
              n182 = while {
                tunnel: w469 -> [w483]
                tunnel: w468 -> [w482]
                tunnel: [w481] -> _
                tunnel: [w480] -> w467
                tunnel: [w475] -> w471
                i -> [w477]
                stop <- w479 stop-if-true
                # "Query Operation Register for new data"
                n183 = Equal?(x="Timeout [ms]", y=w477) -> (x = y?=w476:bool)
                n184 = local read "Stop Measurement"() -> (w474:bool)
                n185 = call "PM100D_Read.vi"("error in (no error)"=w482, "Command"="STAT:OPER?", "VISA in"=w483) -> ("error out"=w480:errorcluster, "ReadValue"=w486:string, "VISA out"=w481:refnum<visa-resource-name>)  [unwired: 1 in]
                n186 = Decimal String To Number(string=w486) -> (number=w485:i32)  [unwired: 2 in, 1 out]
                n187 = Equal?(x=w485, y=512) -> (x = y?=w475:bool)
                "New" <- w475
                n188 = Compound Arithmetic op=OR(w475, w476, w474) -> (w479:bool)
              }
              n189 = Select(t=enum16{"0", "1", "2", "3"}."2", s=w471, f=enum16{"0", "1", "2", "3"}."1") -> (s? t:f=w472:enum16{"0", "1", "2", "3"})
            }
            frame #2 {
              n190 = call "PM100D_Read.vi"("error in (no error)"=w494, "Command"="FETC?", "VISA in"=w495) -> ("error out"=w493:errorcluster, "ReadValue"=w499:string)  [unwired: 1 in, 1 out]
              n191 = Fract/Exp String To Number(use system decimal point (T)=FALSE, string=w499) -> (number=w491:dbl)  [unwired: 2 in, 1 out]
              "Readout value" <- w491
              n192 = Build Array (concatenate)(w490, w491) -> (w489:dbl[])
              "Power Measurement" <- w489
              n193 = Format Into String(format string="%.;%_4p%s", w491, "W" ("Command")) -> (resulting string=→"Readout string":string)  [unwired: 2 in, 1 out]
            }
            frame #3 {
              n194 = local write "Stop Measurement"(TRUE ("t")) -> ()
            }
          }
        }
        n195 = case shown="False" "Save Measurement?" {
          tunnel: w331 -> [_ w340]
          frame #0 {
          }
          frame #1 {
            n196 = call-poly <vilib>:"Write To Spreadsheet File.vi"("transpose? (no:F)"=TRUE, "format (%.3f)"="%#.3e", "1D data"=w340, "file path (dialog if empty)"="Measurement Save Path") -> ()  [unwired: 4 in, 1 out]
          }
        }
        n197 = local read "Scan"() -> (w328:bool)
        n198 = Select(t=7 ("x"), s=w328, f=9 ("x")) -> (s? t:f=w327:i32)
      }
      frame #9 {
        w505 = FALSE
        n199 = local write "Save Current?"(w505) -> ()
        n200 = local write "Measuring Current"(w505) -> ()
        n201 = local write "Current Scan"(w505) -> ()
        n202 = local write "Stop Measurement"(w505) -> ()
        n203 = local write "Save Measurement?"(w505) -> ()
        n204 = local write "Abort\n Scan"(w505) -> ()
        n205 = local write "Save Power Scan?"(w505) -> ()
        n206 = local write "Incrementing Up"(w505) -> ()
        n207 = local write "Scanning"(w505) -> ()
        n208 = local write "Incrementing Down"(w505) -> ()
        n209 = local write "Changing Wavelength"(w505) -> ()
        n210 = local write "Initialize"(w505) -> ()
        n211 = local write "Switch Turret"(w505) -> ()
        n212 = local write "Change Wavelength"(w505) -> ()
        n213 = local write "Increment Up"(w505) -> ()
        n214 = local write "Increment Down"(w505) -> ()
        n215 = local write "Scan"(w505) -> ()
        n216 = local write "Measure Power"(w505) -> ()
        n217 = local write "End Scan"(w505) -> ()
        "Turning Turret" <- w505
      }
      frame #10 {
        w524 = 10178 items=["Finite Samples"=10178, "Continuous Samples"=10123, "Hardware Timed Single Point"=12522] ("sample mode")
        w511 = dbl[] []
        n218 = local read "Ending\nWavelength"() -> (w534:dbl)
        n219 = local read "Starting\nWavelength"() -> (w531:dbl)
        n220 = local read "Wavelength\n   Step Size"() -> (w530:dbl)
        n221 = local read "Step Time (sec)"() -> (w516:dbl)
        n222 = call-poly <vilib>:"DAQmx Create Virtual Channel.vi"("physical channels"="Current") -> ("task out"=w526:refnum<k21>, "error out"=w527:errorcluster)  [unwired: 13 in]
        n223 = case shown="True" "Normalize with file?" {
          tunnel: [dbl[] [] w541] -> w513
          frame #0 {
          }
          frame #1 {
            n224 = call-poly <vilib>:"Read From Spreadsheet File.vi"("transpose (no:F)"=TRUE ("transpose? (no:F)"), "format (%.3f)"="%#.3e", "file path (dialog if empty)"="Open Power Normalization Values Path") -> ("first row"=w541:dbl[])  [unwired: 4 in, 4 out]
          }
        }
        n225 = call-poly <vilib>:"DAQmx Timing.vi"("task/channels in"=w526, "sample mode"=w524, "rate"=250.0, "error in"=w527) -> ("task out"=w515:refnum<k21>, "error out"=w514:errorcluster)  [unwired: 10 in]
        n226 = Subtract(x=w534, y=w531) -> (x-y=w537:dbl)
        n227 = Divide(x=w537, y=w530) -> (x/y=w536:dbl)
        n228 = Round To Nearest(number=w536) -> (nearest integer value=w535:dbl)
        n229 = To Long Integer(number=w535) -> (32bit integer=w533:i32)
        n230 = while {
          tunnel: w533 -> [w576]
          shift-right: [w561] -> w519
          shift-left: w511 -> [w565]
          tunnel: w532 -> [w575]
          tunnel: w531 -> [w572]
          tunnel: w530 -> [w574]
          shift-right: [w570] -> w528
          shift-left: w529 -> [w571]
          shift-right: [w559] -> w518
          shift-left: w511 -> [w566]
          tunnel: w515 -> [w568]
          tunnel: w516 -> [w563]
          tunnel: w514 -> [w562]
          tunnel: w513 -> [w555]
          tunnel: "Normalize with file?" -> [w557]
          shift-right: [w549] -> _
          shift-left: w511 -> [w551]
          i -> [w554]
          stop <- w579 stop-if-true
          n231 = Multiply(x=w554, y=w574) -> (x*y=w573:dbl)
          n232 = Less Or Equal?(x=w576, y=w554) -> (x <= y?=w578:bool)
          n233 = Add(x=w573, y=w572) -> (x+y=w569:dbl)
          n234 = local write "Target\nWavelength"(w569) -> ()
          n235 = Build Array (concatenate)(w551, 1.0 ("element")) -> (w550:dbl[])
          n236 = Build Array (concatenate)(w566, w569) -> (w559:dbl[])
          n237 = Or(x=w578, y="End Scan") -> (x .or. y?=w579:bool)
          n238 = Array Subset(array=w555, index=0, length=w554) -> (w553:dbl[])
          n239 = Select(t=w553, s=w557, f=w550) -> (s? t:f=w549:dbl[])
          n240 = stacked-sequence {
            seq-local: [w580 _ _] -> [_ w585 _]
            tunnel: w575 -> [w583 w587 _]
            tunnel: w569 -> [w582 _ _]
            tunnel: w571 -> [w581 _ _]
            tunnel: [_ w584 _] -> w570
            tunnel: w568 -> [_ _ w599]
            tunnel: [_ _ w596] -> w567
            tunnel: w563 -> [_ _ w594]
            tunnel: w562 -> [_ _ w588]
            frame #0 {
              n241 = call "JYMoveToWavelength.vi"("error in (no error)"=w581, "Target WL"=w582, "RefNum In"=w583) -> ("error out"=w580:errorcluster)  [unwired: 1 in, 2 out]
            }
            frame #1 {
              n242 = call "JYGetCurrentWL.vi"("error in (no error)"=w585, "JYMONOLib.IJYMonoReqd"=w587) -> ("error out"=w584:errorcluster, "Current WL"=w586:dbl)  [unwired: 6 in, 2 out]
              n243 = local write "Wavelength (nm)"(w586) -> ()
            }
            frame #2 {
              n244 = Round To Nearest(number=w594) -> (nearest integer value=w595:dbl)
              n245 = To Long Integer(number=w595) -> (32bit integer=w592:i32)
              n246 = Multiply(x=250 ("number of samples per channel"), y=w592) -> (x*y=w591:i32)
              n247 = call-poly <vilib>:"DAQmx Read.vi"("task/channels in"=w599, "number of samples per channel"=w591, "timeout"=10.0, "error in"=w588) -> ("task out"=w589:refnum<k21>, "data"=w597:dbl[], "error out"=w590:errorcluster)  [unwired: 9 in]
              n248 = call <vilib>:"DAQmx Stop Task.vi"("task/channels in"=w589, "error in"=w590) -> ()  [unwired: 12 in, 2 out]
              n249 = call <vilib>:"Mean.vi"("X"=w597) -> ("mean"=w596:dbl)  [unwired: 1 out]
            }
          }
          n250 = Build Array (concatenate)(w565, w567) -> (w561:dbl[])
          n251 = Divide(x=w561, y=w549) -> (x/y=w560:dbl[])
          n252 = Bundle(w559, w560) -> (→"Normalized Current":cluster{dbl[], dbl[]})  [unwired: 1 in]
          n253 = Bundle(w559, w561) -> (→"Spectral Current":cluster{dbl[], dbl[]})  [unwired: 1 in]
        }
        n254 = Build Array(w519, w518) -> (w517:dbl[][])
        n255 = case shown="True" "Save Current?" {
          tunnel: w517 -> [_ w545]
          frame #0 {
          }
          frame #1 {
            n256 = call-poly <vilib>:"Write To Spreadsheet File.vi"("transpose? (no:F)"=TRUE, "format (%.3f)"="%#.3e", "2D data"=w545, "file path (dialog if empty)"="Save Current Path") -> ()  [unwired: 4 in, 1 out]
          }
        }
        "Measuring Current" <- TRUE ("Scanning")
      }
    }
    "error out" <- w11
  }
  n257 = call "PM100D_Close.vi"("error in (no error)"=w3, "VISA resource name"=w2) -> ()  [unwired: 2 in]
  n258 = local write "Status"("Disconnected...") -> ()
  n259 = local write "Exit"(w1) -> ()
  n260 = local write "Initialized"(w1) -> ()
